vi "LlenarTabla.vi"(8 "error in (no error)":errorcluster, 11 "Prueba32 in":refnum<class "Prueba32.lvclass">) -> (0 "error out":errorcluster, 3 "Prueba32 out":refnum<class "Prueba32.lvclass">)   [LabVIEW 2019, in "Prueba32.lvclass"]
uses:
  Prueba32.lvclass
  Prueba32.lvclass/Prueba32.ctl
panel:
  out "Tabla_Int":string[][](table)
  out "Tabla_Ext":string[][](table)=[["63"], ["125"], ["250"], ["500"], ["1000"], ["2000"], ["4000"], ["8000"]]
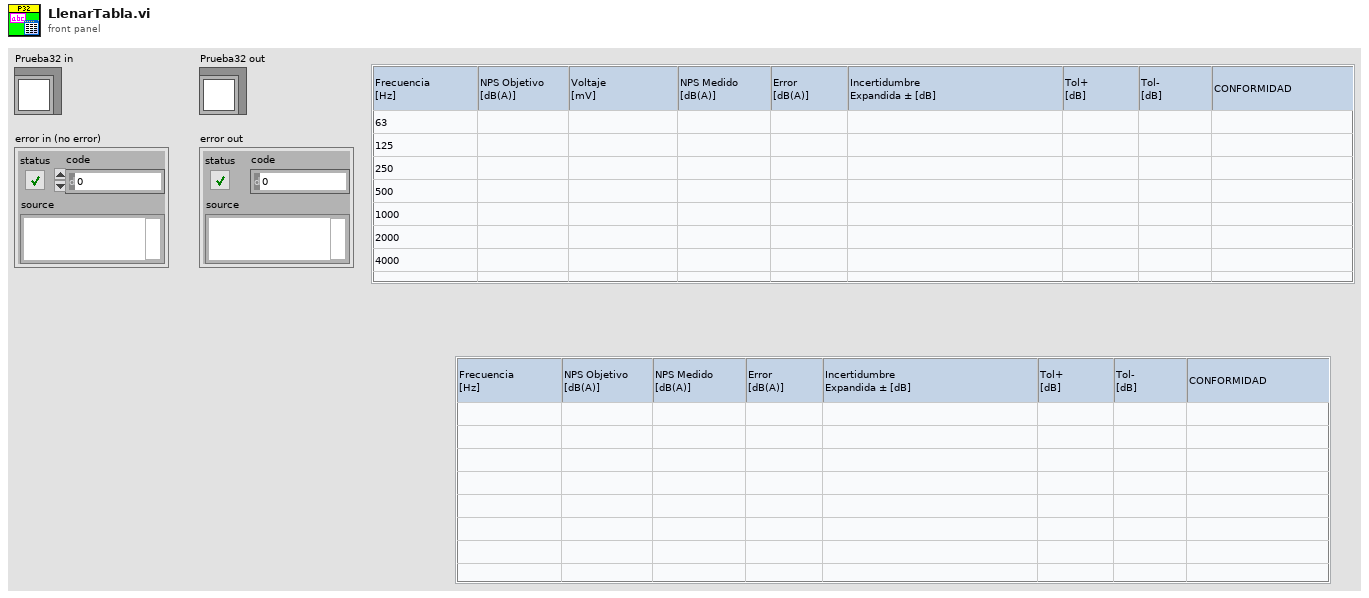
[diagram p1: front panel]
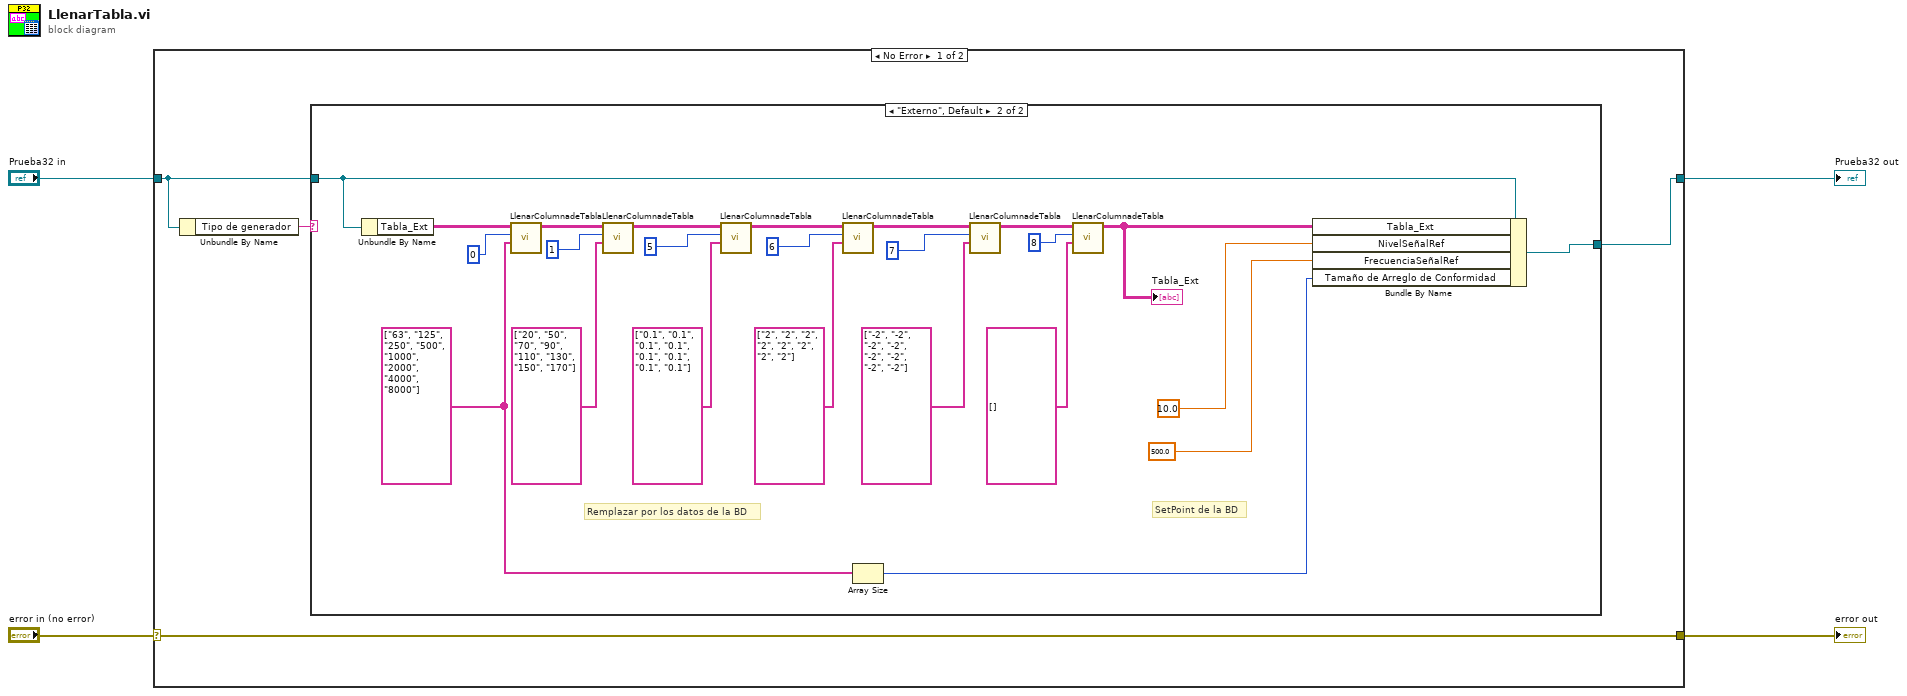
[diagram p0: block diagram]
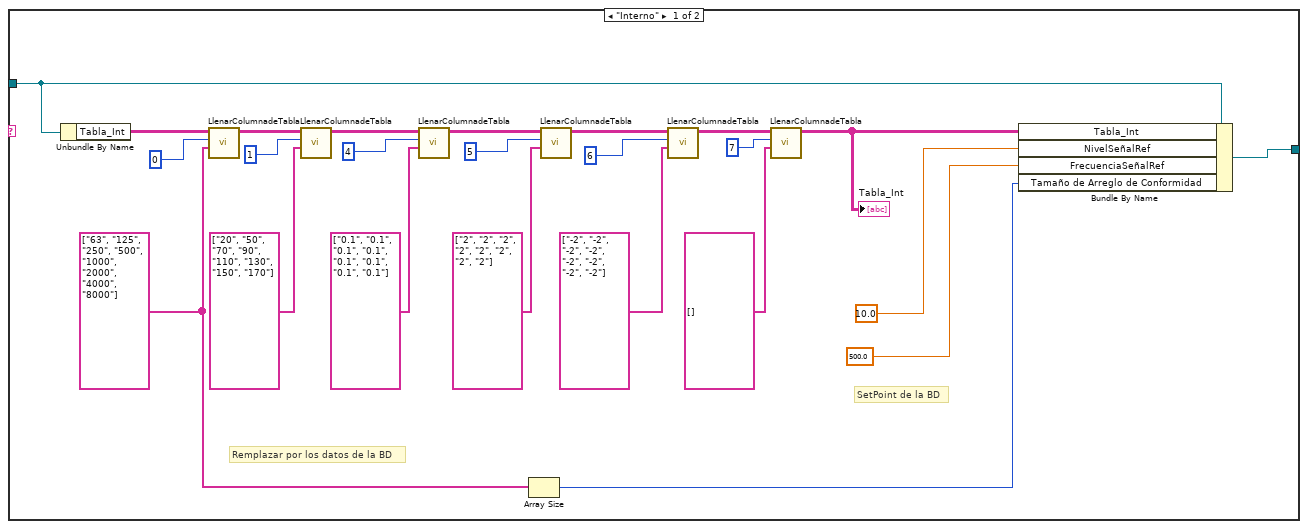
[diagram p2: hidden frame]
diagram:
  n1 = case shown="No Error" "error in (no error)" {
    selector: "error in (no error)" -> [w8 w57]
    tunnel: [w8 w57] -> w2
    tunnel: [w7 w58] -> w3
    tunnel: "Prueba32 in" -> [w6 w58]
    frame No Error {
      n2 = Unbundle By Name(w6) -> ("Tipo de generador"=w5:string)
      n3 = case shown="\"Externo\", Default" w5 {
        tunnel: [w31 w55] -> w7
        tunnel: w6 -> [w30 w54]
        frame "Interno" {
          w11 = string[] ["63", "125", "250", "500", "1000", "2000", "4000", "8000"]
          # "SetPoint de la BD"
          # "Remplazar por los datos de la BD"
          n4 = Unbundle By Name(w30) -> ("Tabla_Int"=w32:string[][])
          n5 = call "LlenarColumnadeTabla.vi"("Data"=w11, "Col. Number"=0, "Tabla in"=w32) -> ("Tabla out"=w28:string[][])  [unwired: 8 in]
          n6 = call "LlenarColumnadeTabla.vi"("Data"=string[] ["20", "50", "70", "90", "110", "130", "150", "170"], "Col. Number"=1, "Tabla in"=w28) -> ("Tabla out"=w18:string[][])  [unwired: 8 in]
          n7 = call "LlenarColumnadeTabla.vi"("Data"=string[] ["0.1", "0.1", "0.1", "0.1", "0.1", "0.1", "0.1", "0.1"], "Col. Number"=4, "Tabla in"=w18) -> ("Tabla out"=w17:string[][])  [unwired: 8 in]
          n8 = Array Size(array=w11) -> (size(s)=w10:i32)
          n9 = call "LlenarColumnadeTabla.vi"("Data"=string[] ["2", "2", "2", "2", "2", "2", "2", "2"], "Col. Number"=5, "Tabla in"=w17) -> ("Tabla out"=w25:string[][])  [unwired: 8 in]
          n10 = call "LlenarColumnadeTabla.vi"("Data"=string[] ["-2", "-2", "-2", "-2", "-2", "-2", "-2", "-2"], "Col. Number"=6, "Tabla in"=w25) -> ("Tabla out"=w14:string[][])  [unwired: 8 in]
          n11 = call "LlenarColumnadeTabla.vi"("Data"=string[] [], "Col. Number"=7, "Tabla in"=w14) -> ("Tabla out"=w9:string[][])  [unwired: 8 in]
          "Tabla_Int" <- w9
          n12 = Bundle By Name(cluster=w30, "Tabla_Int"=w9, "NivelSeñalRef"=10.0, "FrecuenciaSeñalRef"=500.0, "Tamaño de Arreglo de Conformidad"=w10) -> (w31:refnum<class "Prueba32.lvclass">)
        }
        frame "Externo", Default {
          w35 = string[] ["63", "125", "250", "500", "1000", "2000", "4000", "8000"]
          # "SetPoint de la BD"
          # "Remplazar por los datos de la BD"
          n13 = Unbundle By Name(w54) -> ("Tabla_Ext"=w56:string[][])
          n14 = call "LlenarColumnadeTabla.vi"("Data"=w35, "Col. Number"=0, "Tabla in"=w56) -> ("Tabla out"=w52:string[][])  [unwired: 8 in]
          n15 = call "LlenarColumnadeTabla.vi"("Data"=string[] ["20", "50", "70", "90", "110", "130", "150", "170"], "Col. Number"=1, "Tabla in"=w52) -> ("Tabla out"=w42:string[][])  [unwired: 8 in]
          n16 = call "LlenarColumnadeTabla.vi"("Data"=string[] ["0.1", "0.1", "0.1", "0.1", "0.1", "0.1", "0.1", "0.1"], "Col. Number"=5, "Tabla in"=w42) -> ("Tabla out"=w41:string[][])  [unwired: 8 in]
          n17 = call "LlenarColumnadeTabla.vi"("Data"=string[] ["2", "2", "2", "2", "2", "2", "2", "2"], "Col. Number"=6, "Tabla in"=w41) -> ("Tabla out"=w49:string[][])  [unwired: 8 in]
          n18 = Array Size(array=w35) -> (size(s)=w34:i32)
          n19 = call "LlenarColumnadeTabla.vi"("Data"=string[] ["-2", "-2", "-2", "-2", "-2", "-2", "-2", "-2"], "Col. Number"=7, "Tabla in"=w49) -> ("Tabla out"=w38:string[][])  [unwired: 8 in]
          n20 = call "LlenarColumnadeTabla.vi"("Data"=string[] [], "Col. Number"=8, "Tabla in"=w38) -> ("Tabla out"=w33:string[][])  [unwired: 8 in]
          "Tabla_Ext" <- w33
          n21 = Bundle By Name(cluster=w54, "Tabla_Ext"=w33, "NivelSeñalRef"=10.0, "FrecuenciaSeñalRef"=500.0, "Tamaño de Arreglo de Conformidad"=w34) -> (w55:refnum<class "Prueba32.lvclass">)
        }
      }
    }
    frame Error {
    }
  }
  "Prueba32 out" <- w3
  "error out" <- w2
